vi "共享变量发布.vi"() -> ()   [LabVIEW 2016]
panel:
  in  "数组":cluster{"IP":string, "port":i32}[](array[cluster])
  out "变体":variant
  out "错误输出":errorcluster
  in  "停止":bool
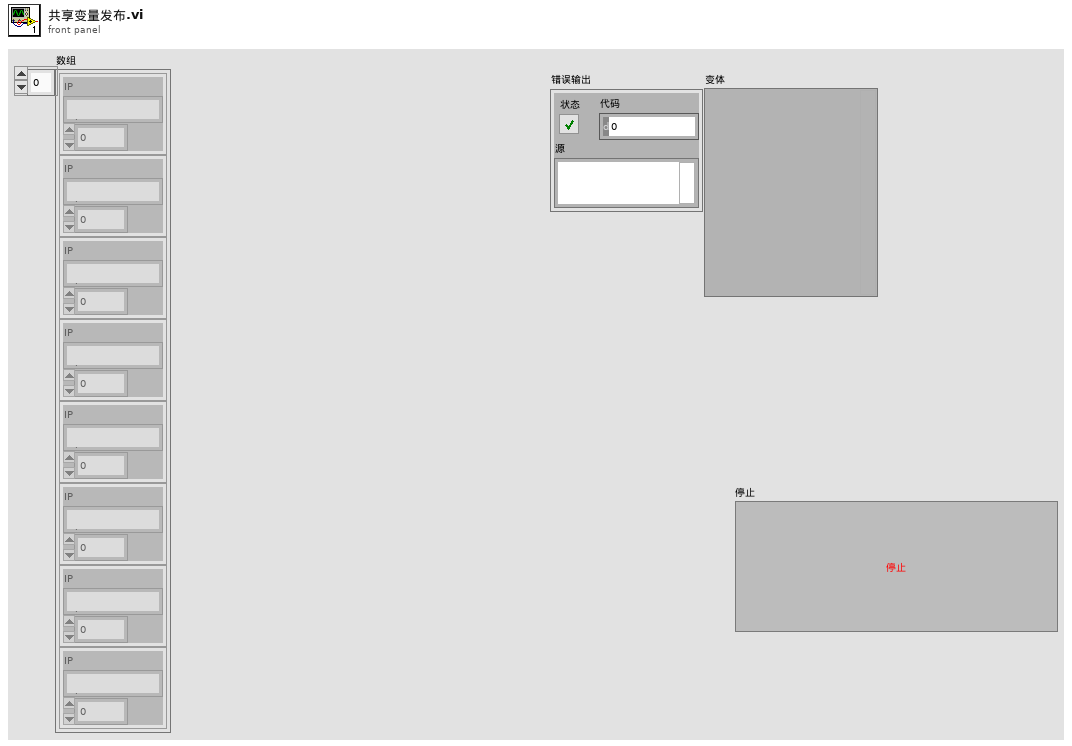
[diagram p1: front panel]
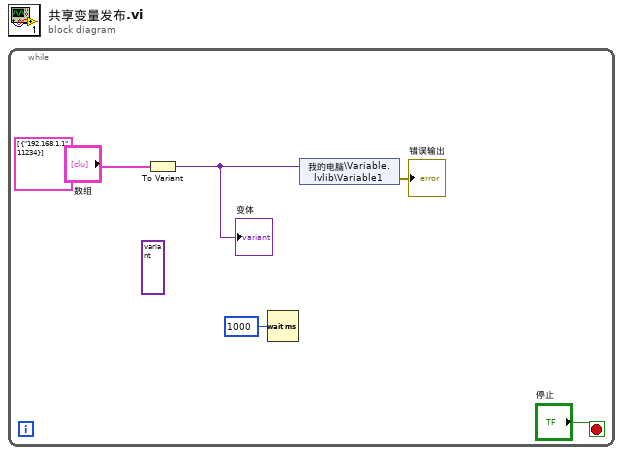
[diagram p0: block diagram]
diagram:
  n1 = while {
    stop <- "停止" stop-if-true
    (unwired) cluster{"IP":string, "port":i32}[] [{"IP"="192.168.1.1", "port"=11234}] ("数组")
    (unwired) variant(cluster{"IP":string, "port":i32}[] []) ("变体")
    n2 = To Variant(anything="数组") -> (Variant=w2:variant)
    "变体" <- w2
    n3 = Wait (ms)(milliseconds to wait=u32 1000 ("等待时间（毫秒）")) -> ()  [unwired: 1 out]
    n4 = shared-variable "我的电脑\\Variable.lvlib\\Variable1"(w2) -> (error out=→"错误输出":errorcluster)  [unwired: 1 in]
  }
